vi "Set Initialization Data - ChartView.vi"(8 "error in":errorcluster, 11 "Manager Worker in":refnum<class "Manager Worker.lvclass">) -> (0 "error out":errorcluster, 3 "Manager Worker out":refnum<class "Manager Worker.lvclass">)   [LabVIEW 2018, in "Manager Worker.lvclass"]
doc: "Sets the initialization data of a statically linked subWorker."
uses:
  Manager Worker.lvclass
  ChartView Worker/Initialization Data.ctl
  <vilib>/addons/_Workers/Library/Classes/Message Queue/Message Queue.lvclass
  Manager Worker.lvclass/Manager Worker.ctl
  <vilib>/addons/_Workers/Library/Classes/Worker/Worker.lvclass/Worker.ctl
  <vilib>/addons/_Workers/Library/Classes/Worker/Read Queue.vi
  Acquire Worker/DataAcquire Worker.lvclass
  D:/Program Files (x86)/National Instruments/LabVIEW 2018/vi.lib/addons/_Workers/Library/Classes/Worker/Worker.lvclass
  ChartView Worker/ChartView Worker.lvclass
  <vilib>/addons/_Workers/Library/Classes/Worker/Worker.lvclass
  D:/Program Files (x86)/National Instruments/LabVIEW 2018/vi.lib/addons/_Workers/Library/Classes/Workers Object/Workers Object.lvclass
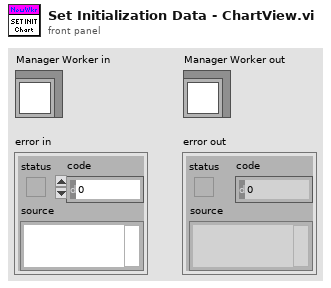
[diagram p1: front panel]
types:
  T1 = typedef "ChartView Worker.lvclass/Initialization Data.ctl" = cluster{"String":string, "Acquire Queue":refnum<class "Message Queue.lvclass">}
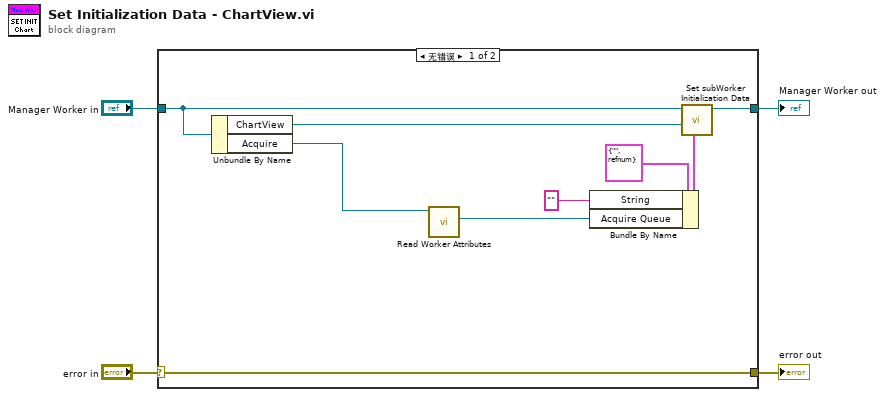
[diagram p0: block diagram]
diagram:
  n1 = case shown="无错误" "error in" {
    selector: "error in" -> [w13 w15]
    tunnel: [w13 w15] -> w3
    tunnel: [w11 w14] -> w2
    tunnel: "Manager Worker in" -> [w10 w14]
    frame No Error {
      n2 = Unbundle By Name(w10) -> ("ChartView"=w12:refnum<class "ChartView Worker.lvclass">, "Acquire"=w6:refnum<class "DataAcquire Worker.lvclass">)
      n3 = call-poly <vilib>:"Read Worker Attributes.vi"("Worker"=w6) -> ("Message Queue out"=w5:refnum<class "Message Queue.lvclass">)  [unwired: 9 in, 1 out]
      n4 = Bundle By Name(cluster=T1 {"String"="", "Acquire Queue"=refnum} ("Initialization Data"), "String"="" ("Placeholder"), "Acquire Queue"=w5) -> (w8:T1)
      n5 = call-dynamic "Set subWorker Initialization Data.vi"("Initialization Data"=w8, "subWorker"=w12, "Worker"=w10) -> ("Worker out"=w11:refnum<class "Manager Worker.lvclass">)  [unwired: 8 in]
    }
    frame Error {
    }
  }
  "error out" <- w3
  "Manager Worker out" <- w2
